vi "configureTrigger_action.vi"(0 "HGF_Basler_A602f":refnum<class "HGF_Basler_A602f.lvclass">, 1 "Type":u32(ring) items=["External"=0, "RTSI"=1, "ISO In"=2, "Scaled Encoder"=5, "Software Trigger"=6], 2 "Line Number":u32, 3 "Frame timeout (ms)":u32=1000, 4 "Action":u32(ring) items=["Disabled", "Trigger start of acquisition", "Trigger start of each buffer list", "Trigger each buffer", "Trigger each line (linescan)", "Trigger end of acquisition"], 5 "error in (no error)":errorcluster, 6 "Activation":u32(ring) items=["Rising Edge", "Falling Edge", "AnyEdge", "LevelHigh", "LevelLow"], 7 "Delay":cluster{"Value":dbl, "Units":u32}={"Value"=0.0, "Units"=5} {"Units" items=["Scaled Encoder Counts"=4, "Milliseconds"=5]}, 8 "Mode":T1(ring), 9 "Skip trigger (linescan only)":u32) -> (14 "dup HGF_Basler_A602f":refnum<class "HGF_Basler_A602f.lvclass">, 19 "error out":errorcluster)   [LabVIEW 2014, in "HGF_IMAQ.lvlib" / "HGF_Basler_A602f.lvclass"]
doc: "Configures the trigger conditions for an acquisition. Use this VI before any acquisition VI to setup a triggered image acquisition."
uses:
  HGF_Basler_A602f.lvclass
  VisionTools/HGF_VisionTools/HGF_VisionTools.lvlib
  VisionTools/HGF_VisionTools/IMAQdx_setAttribute_Enum.vi
  HGF_Auxiliary/ErrorCode.ctl
  HGF_Auxiliary/HGF_Auxiliary.lvlib
  HGF_Auxiliary/Severity.ctl
  HGF_ImaqDx/HGF_ImaqDx.lvclass
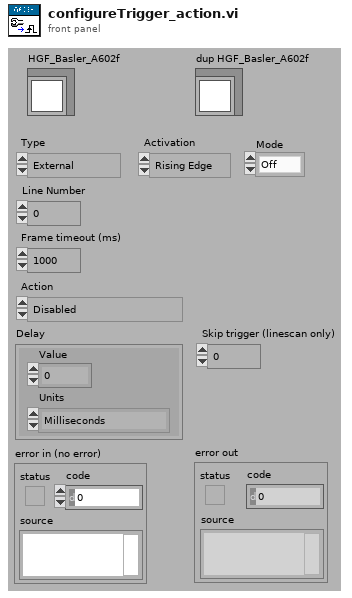
[diagram p1: front panel]
types:
  T1 = enum16{"Off", "Mode 0", "Mode 1", "Mode 2", "Mode 3", "Mode 4", "Mode 5"}
  T2 = typedef "HGF_Auxiliary.lvlib/Severity.ctl" = enum16{"Info", "Warning", "Fault", "Error", "Fatal"}
  T3 = typedef "HGF_Auxiliary.lvlib/ErrorCode.ctl" = enum32{"No error", "Function not supported.", "This VI is for friends only.", "Reference object aready exisits.", "Parameter out of range.", "Not a rendezvous.", "Invalid notifier reference.", "Invalid queue reference.", "Self-Test not supported.", "Reset not supported.", "IDN query not supported.", "Error query not supported.", "Incorrect addressee.", "Object already exists.", "No class name specified", "Driver not supported", "Attribute is not writable"}
  T4 = typedef "IMAQdx.ctl" = refnum<k21>
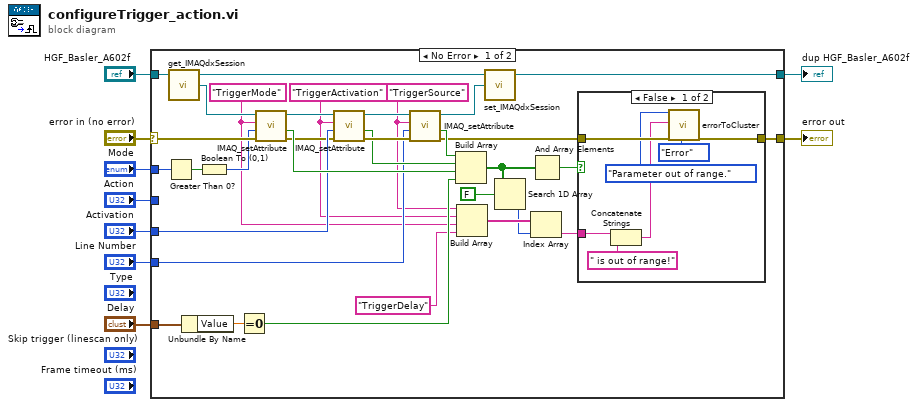
[diagram p0: block diagram]
diagram:
  n1 = case shown="No Error" "error in (no error)" {
    selector: "error in (no error)" -> [w40 w51]
    tunnel: "HGF_Basler_A602f" -> [w28 w52]
    tunnel: [w36 w51] -> w7
    tunnel: [w26 w52] -> w8
    tunnel: "Activation" -> [w34 _]
    tunnel: "Mode" -> [w33 _]
    tunnel: "Line Number" -> [w30 _]
    tunnel: "Action" -> [_ _]
    tunnel: "Delay" -> [w22 _]
    frame No Error {
      w12 = "TriggerSource" ("Attribute Name")
      w11 = "TriggerActivation" ("Attribute Name")
      w10 = "TriggerMode" ("Attribute Name")
      n2 = Greater Than 0?(x=w33) -> (x > 0?=w32:bool)
      n3 = call "get_IMAQdxSession.vi"("HGF_ImaqDx in"=w28) -> ("IMAQdx Session"=w29:T4, "HGF_ImaqDx out"=w27:refnum<class "HGF_Basler_A602f.lvclass">)  [unwired: 2 in, 1 out]
      n4 = Unbundle By Name(w22) -> ("Value"=w21:dbl)
      n5 = Boolean To (0,1)(Boolean=w32) -> (0, 1=w31:i16)
      n6 = Equal To 0?(x=w21) -> (x = 0?=w20:bool)
      n7 = call-poly "IMAQ_setAttribute.vi"("error in (no error)"=w40, "Value (Enum)"=w31, "Attribute Name"=w10, "IMAQdx Session"=w29) -> ("error out"=w23:errorcluster, "In Range?"=w37:bool, "dup IMAQdx Session"=w24:T4)  [unwired: 1 in]
      n8 = call-poly "IMAQ_setAttribute.vi"("error in (no error)"=w23, "Value (Enum)"=w34, "Attribute Name"=w11, "IMAQdx Session"=w24) -> ("error out"=w42:errorcluster, "In Range?"=w38:bool, "dup IMAQdx Session"=w41:T4)  [unwired: 1 in]
      n9 = call-poly "IMAQ_setAttribute.vi"("error in (no error)"=w42, "Value (Enum)"=w30, "Attribute Name"=w12, "IMAQdx Session"=w41) -> ("error out"=w35:errorcluster, "In Range?"=w39:bool, "dup IMAQdx Session"=w25:T4)  [unwired: 1 in]
      n10 = Build Array(w39, w38, w37, w20) -> (w18:bool[])
      n11 = Build Array(w12, w11, w10, "TriggerDelay" ("element")) -> (w16:string[])
      n12 = call "set_IMAQdxSession.vi"("IMAQdx Session"=w25, "HGF_ImaqDx in"=w27) -> ("HGF_ImaqDx out"=w26:refnum<class "HGF_Basler_A602f.lvclass">)  [unwired: 2 in, 1 out]
      n13 = Search 1D Array(1D array=w18, element=FALSE) -> (index of element=w15:i32)  [unwired: 1 in]
      n14 = Index Array(array=w16, index=w15) -> (element=w13:string)
      n15 = And Array Elements(Boolean array=w18) -> (logical AND=w19:bool)
      n16 = case shown="False" w19 {
        tunnel: w35 -> [w49 w50]
        tunnel: [w48 w50] -> w36
        tunnel: w13 -> [w44 _]
        frame False {
          n17 = Concatenate Strings(w44, " is out of range!" ("string")) -> (w43:string)
          n18 = call "errorToCluster.vi"("error code"=ErrorCode."Parameter out of range.", "error message (\"\")"=w43, "error in (no error)"=w49, "severity (Error)"=Severity."Error") -> ("error out"=w48:errorcluster)  [unwired: 15 in]
        }
        frame True {
        }
      }
    }
    frame Error {
    }
  }
  "error out" <- w7
  "dup HGF_Basler_A602f" <- w8
